vi "Read Registers.vi"(8 "error in (no error)":errorcluster, 11 "Serial Config":T3={"设备名称"="", "串口选择"="COM1", "仪器地址"=200, "通讯速率"=8, "超时时间"=0, "刷新时间"=10.0}) -> (0 "error out":errorcluster, 1 "DecimalPoint2":i16, 2 "Response List":T1[](array[typedef]), 3 "DecimalPoint1":i16, 4 "SP 2":dbl format="%.2f", 5 "Input2 Value":dbl format="%.2f", 6 "SP 1":dbl format="%.2f", 7 "Input1 Value":dbl format="%.2f")   [LabVIEW 2010, in "MonitorServer.lvlib"]
uses:
  MonitorServer.lvlib
  Serial Config.ctl
  SubVIs/ModBUS Driver/Private/MBDRV_Response.ctl
  SubVIs/ModBUS Driver/Private/MBDRV_Action.ctl
  SubVIs/ModBUS Driver/Private/MBDRV_Command List.ctl
  SubVIs/ModBUS Driver/Private/MBDRV_Command Data.ctl
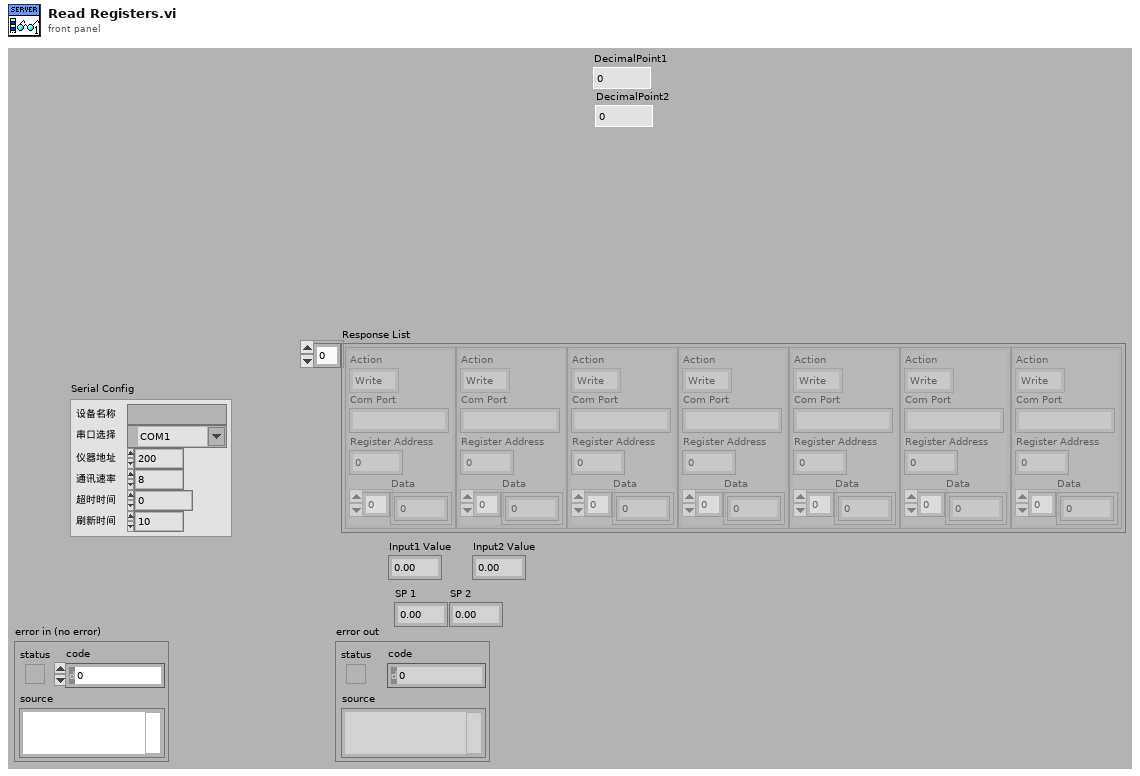
[diagram p1: front panel]
types:
  T1 = typedef "MBDRV_Response.ctl" = cluster{"Action":T2, "Com Port":string, "Register Address":u16, "Data":i16[]}
  T2 = typedef "MBDRV_Action.ctl" = enum16{"Write", "Read"}
  T3 = typedef "MonitorServer.lvlib/Serial Config.ctl" = cluster{"设备名称":string, "串口选择":refnum<visa-resource-name>, "仪器地址":u32, "通讯速率":u32, "超时时间":u32, "刷新时间":dbl}
  T4 = typedef "MBDRV_Command List.ctl" = T5[]
  T5 = typedef "MBDRV_Command Data.ctl" = cluster{"Action":T2, "Com Port":string, "Register Address":u16, "Data To Write/Num To Read":i16}
  T6 = typedef "MBDRV_Response List.ctl" = T1[]
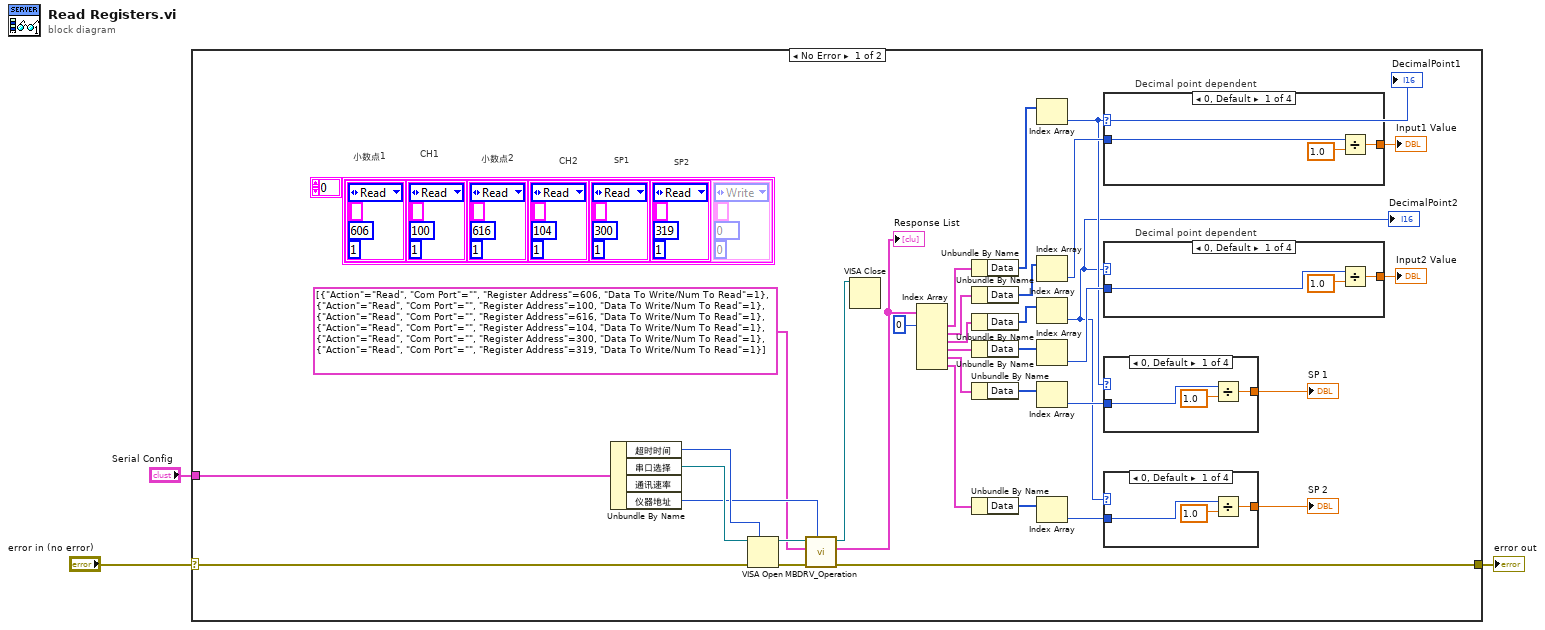
[diagram p0: block diagram]
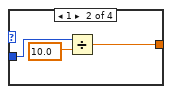
[diagram p2: hidden frame]
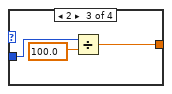
[diagram p3: hidden frame]
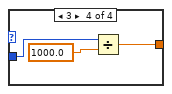
[diagram p4: hidden frame]
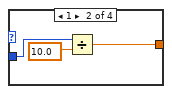
[diagram p5: hidden frame]
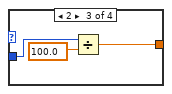
[diagram p6: hidden frame]
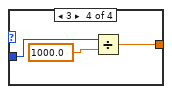
[diagram p7: hidden frame]
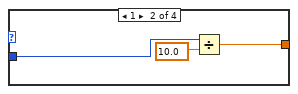
[diagram p8: hidden frame]
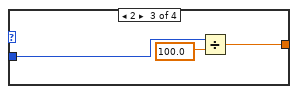
[diagram p9: hidden frame]
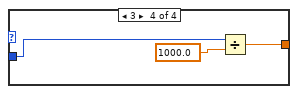
[diagram p10: hidden frame]
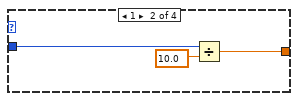
[diagram p11: hidden frame]
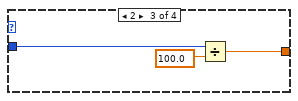
[diagram p12: hidden frame]
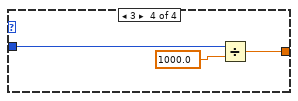
[diagram p13: hidden frame]
diagram:
  n1 = case shown="No Error" "error in (no error)" {
    selector: "error in (no error)" -> [w34 w86]
    tunnel: "Serial Config" -> [w35 _]
    tunnel: [w30 w86] -> w1
    frame No Error {
      # "SP2"
      # "SP1"
      # "CH2"
      # "小数点2"
      # "CH1"
      # "小数点1"
      # "Decimal point dependent"
      # "Decimal point dependent"
      n2 = Unbundle By Name(w35) -> ("超时时间"=w36:u32, "串口选择"=w37:refnum<visa-resource-name>, "仪器地址"=w32:u32)  [unwired: 1 out]
      n3 = VISA Open(timeout (0)=w36, error in (no error)=w34, VISA resource name=w37) -> (VISA resource name=w33:refnum<visa-resource-name>, error out=w31:errorcluster)  [unwired: 2 in]
      n4 = call "MBDRV_Operation.vi"("Unit Address (1)"=w32, "error in (no error)"=w31, "Command List"=T4 [{"Action"=enum."Read", "Com Port"="", "Register Address"=606, "Data To Write/Num To Read"=1}, {"Action"=enum."Read", "Com Port"="", "Register Address"=100, "Data To Write/Num To Read"=1}, {"Action"=enum."Read", "Com Port"="", "Register Address"=616, "Data To Write/Num To Read"=1}, {"Action"=enum."Read", "Com Port"="", "Register Address"=104, "Data To Write/Num To Read"=1}, {"Action"=enum."Read", "Com Port"="", "Register Address"=300, "Data To Write/Num To Read"=1}, {"Action"=enum."Read", "Com Port"="", "Register Address"=319, "Data To Write/Num To Read"=1}], "VISA resource name"=w33) -> ("error out"=w30:errorcluster, "Response List"=w28:T6, "VISA resource name out"=w10:refnum<visa-resource-name>)  [unwired: 5 in]
      "Response List" <- w28
      n5 = VISA Close(VISA resource name=w10) -> ()  [unwired: 1 in, 1 out]
      n6 = Index Array(array=w28, index #1=0 ("index")) -> (element #1=w27:T1, element #2=w23:T1, element #3=w16:T1, element #4=w15:T1, element #5=w13:T1, element #6=w12:T1)  [unwired: 5 in]
      n7 = Unbundle By Name(w27) -> ("Data"=w25:i16[])
      n8 = Unbundle By Name(w23) -> ("Data"=w24:i16[])
      n9 = Unbundle By Name(w16) -> ("Data"=w17:i16[])
      n10 = Unbundle By Name(w15) -> ("Data"=w18:i16[])
      n11 = Unbundle By Name(w13) -> ("Data"=w11:i16[])
      n12 = Unbundle By Name(w12) -> ("Data"=w14:i16[])
      n13 = Index Array(array=w25) -> (element=w8:i16)  [unwired: 1 in]
      "DecimalPoint1" <- w8
      n14 = Index Array(array=w24) -> (element=w21:i16)  [unwired: 1 in]
      n15 = Index Array(array=w17) -> (element=w4:i16)  [unwired: 1 in]
      "DecimalPoint2" <- w4
      n16 = Index Array(array=w18) -> (element=w20:i16)  [unwired: 1 in]
      n17 = Index Array(array=w11) -> (element=w7:i16)  [unwired: 1 in]
      n18 = Index Array(array=w14) -> (element=w5:i16)  [unwired: 1 in]
      n19 = case shown="0, Default" w8 {
        tunnel: [w75 w78 w81 w84] -> w22
        tunnel: w21 -> [w74 w77 w80 w83]
        frame 0, Default {
          n20 = Divide(x=w74, y=1.0) -> (x/y=w75:dbl)
        }
        frame 1 {
          n21 = Divide(x=w77, y=10.0) -> (x/y=w78:dbl)
        }
        frame 2 {
          n22 = Divide(x=w80, y=100.0) -> (x/y=w81:dbl)
        }
        frame 3 {
          n23 = Divide(x=w83, y=1000.0) -> (x/y=w84:dbl)
        }
      }
      "Input1 Value" <- w22
      n24 = case shown="0, Default" w4 {
        tunnel: [w63 w66 w69 w72] -> w19
        tunnel: w20 -> [w62 w65 w68 w71]
        frame 0, Default {
          n25 = Divide(x=w62, y=1.0) -> (x/y=w63:dbl)
        }
        frame 1 {
          n26 = Divide(x=w65, y=10.0) -> (x/y=w66:dbl)
        }
        frame 2 {
          n27 = Divide(x=w68, y=100.0) -> (x/y=w69:dbl)
        }
        frame 3 {
          n28 = Divide(x=w71, y=1000.0) -> (x/y=w72:dbl)
        }
      }
      "Input2 Value" <- w19
      n29 = case shown="0, Default" w8 {
        tunnel: [w51 w54 w57 w60] -> w9
        tunnel: w7 -> [w50 w53 w56 w59]
        frame 0, Default {
          n30 = Divide(x=w50, y=1.0) -> (x/y=w51:dbl)
        }
        frame 1 {
          n31 = Divide(x=w53, y=10.0) -> (x/y=w54:dbl)
        }
        frame 2 {
          n32 = Divide(x=w56, y=100.0) -> (x/y=w57:dbl)
        }
        frame 3 {
          n33 = Divide(x=w59, y=1000.0) -> (x/y=w60:dbl)
        }
      }
      "SP 1" <- w9
      n34 = case shown="0, Default" w4 {
        tunnel: [w39 w42 w45 w48] -> w6
        tunnel: w5 -> [w38 w41 w44 w47]
        frame 0, Default {
          n35 = Divide(x=w38, y=1.0) -> (x/y=w39:dbl)
        }
        frame 1 {
          n36 = Divide(x=w41, y=10.0) -> (x/y=w42:dbl)
        }
        frame 2 {
          n37 = Divide(x=w44, y=100.0) -> (x/y=w45:dbl)
        }
        frame 3 {
          n38 = Divide(x=w47, y=1000.0) -> (x/y=w48:dbl)
        }
      }
      "SP 2" <- w6
    }
    frame Error {
    }
  }
  "error out" <- w1
